vi "readmeBD.vi"() -> ()   [LabVIEW 2019]
uses:
  b0a80b8d-123d-4e48-8a3b-454a52138259.vi
  e28731c3-b8ec-45ff-9a0c-526a81498bbc.vi
  ad491d61-f5a4-4c52-8db8-1c7fdc49d802.vi
  LV Colormap Names.ctl
panel:
  in  "Colormap By Name":string="gist_stern"
  in  "Colormap Name (detached enum)":T1(ring)=enum."inferno"
  in  "Colormap Name (original enum)":T2=enum."turbo"
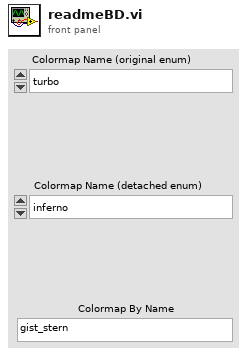
[diagram p1: front panel]
types:
  T1 = enum16{"magma", "inferno", "plasma", "viridis", "cividis", "twilight", "twilight_shifted", "turbo", "berlin", "managua", "vanimo"}
  T2 = typedef "LV Colormap Names.ctl" = enum16{"Accent", "Accent_r", "Blues", "Blues_r", "BrBG", "BrBG_r", "BuGn", "BuGn_r", "BuPu", "BuPu_r", "CMRmap", "CMRmap_r", "Dark2", "Dark2_r", "GnBu", "GnBu_r", "Grays", "Grays_r", "Greens", "Greens_r", "Greys", "Greys_r", "OrRd", "OrRd_r", "Oranges", "Oranges_r", "PRGn", "PRGn_r", "Paired", "Paired_r", "Pastel1", "Pastel1_r", "Pastel2", "Pastel2_r", "PiYG", "PiYG_r", "PuBu", "PuBuGn", "PuBuGn_r", "PuBu_r", "PuOr", "PuOr_r", "PuRd", "PuRd_r", "Purples", "Purples_r", "RdBu", "RdBu_r", "RdGy", "RdGy_r", "RdPu", "RdPu_r", "RdYlBu", "RdYlBu_r", "RdYlGn", "RdYlGn_r", "Reds", "Reds_r", "Set1", "Set1_r", "Set2", "Set2_r", "Set3", "Set3_r", "Spectral", "Spectral_r", "Wistia", "Wistia_r", "YlGn", "YlGnBu", "YlGnBu_r", "YlGn_r", "YlOrBr", "YlOrBr_r", "YlOrRd", "YlOrRd_r", "afmhot", "afmhot_r", "autumn", "autumn_r", "berlin", "berlin_r", "binary", "binary_r", "bone", "bone_r", "brg", "brg_r", "bwr", "bwr_r", "cividis", "cividis_r", "cool", "cool_r", "coolwarm", "coolwarm_r", "copper", "copper_r", "cubehelix", "cubehelix_r", "flag", "flag_r", "gist_earth", "gist_earth_r", "gist_gray", "gist_gray_r", "gist_grey", "gist_grey_r", "gist_heat", "gist_heat_r", "gist_ncar", "gist_ncar_r", "gist_rainbow", "gist_rainbow_r", "gist_stern", "gist_stern_r", "gist_yarg", "gist_yarg_r", "gist_yerg", "gist_yerg_r", "gnuplot", "gnuplot2", "gnuplot2_r", "gnuplot_r", "gray", "gray_r", "grey", "grey_r", "hot", "hot_r", "hsv", "hsv_r", "inferno", "inferno_r", "jet", "jet_r", "magma", "magma_r", "managua", "managua_r", "nipy_spectral", "nipy_spectral_r", "ocean", "ocean_r", "pink", "pink_r", "plasma", "plasma_r", "prism", "prism_r", "rainbow", "rainbow_r", "seismic", "seismic_r", "spring", "spring_r", "summer", "summer_r", "tab10", "tab10_r", "tab20", "tab20_r", "tab20b", "tab20b_r", "tab20c", "tab20c_r", "terrain", "terrain_r", "turbo", "turbo_r", "twilight", "twilight_r", "twilight_shifted", "twilight_shifted_r", "vanimo", "vanimo_r", "viridis", "viridis_r", "winter", "winter_r"}
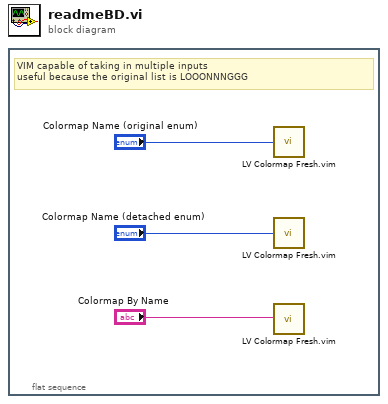
[diagram p0: block diagram]
diagram:
  n1 = flat-sequence {
    frame #0 {
      # "VIM capable of taking in multiple inputs\nuseful because the original list is LOOONNNGGG"
      n2 = call "LV Colormap Fresh.vim"("Colormap Name"="Colormap Name (original enum)") -> ()  [unwired: 14 in, 1 out]
      n3 = call "LV Colormap Fresh.vim"("Colormap Name"="Colormap Name (detached enum)") -> ()  [unwired: 14 in, 1 out]
      n4 = call "LV Colormap Fresh.vim"("Colormap Name"="Colormap By Name") -> ()  [unwired: 14 in, 1 out]
    }
  }
